vi "close.binary.refs.vi"(8 "error in":errorcluster, 11 "binary references":T1) -> (0 "error out":errorcluster)   [LabVIEW 2024, in "manager_daemon.lvclass"]
uses:
  manager_daemon.lvclass
  binary.references--cluster.ctl
  manager_daemon.lvclass/manager_daemon.ctl
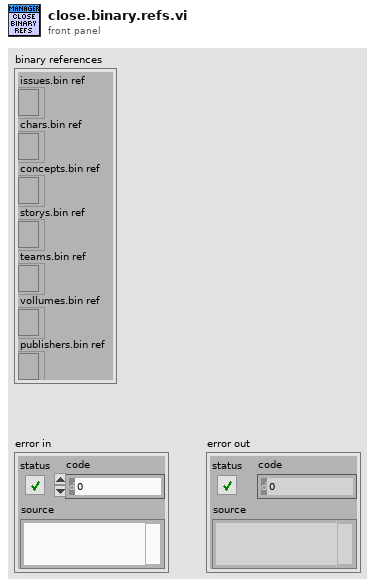
[diagram p1: front panel]
types:
  T1 = typedef "manager_daemon.lvclass/binary.references--cluster.ctl" = cluster{"issues.bin ref":refnum<file>, "chars.bin ref":refnum<file>, "concepts.bin ref":refnum<file>, "storys.bin ref":refnum<file>, "teams.bin ref":refnum<file>, "vollumes.bin ref":refnum<file>, "publishers.bin ref":refnum<file>}
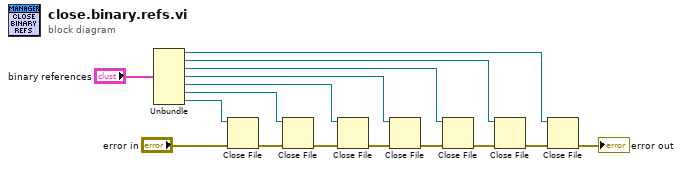
[diagram p0: block diagram]
diagram:
  n1 = Unbundle("binary references") -> ("issues.bin ref"=w3:refnum<file>, "chars.bin ref"=w4:refnum<file>, "concepts.bin ref"=w5:refnum<file>, "storys.bin ref"=w6:refnum<file>, "teams.bin ref"=w7:refnum<file>, "vollumes.bin ref"=w8:refnum<file>, "publishers.bin ref"=w15:refnum<file>)
  n2 = Close File(refnum=w15, error in="error in") -> (error out=w11:errorcluster)  [unwired: 1 out]
  n3 = Close File(refnum=w8, error in=w11) -> (error out=w14:errorcluster)  [unwired: 1 out]
  n4 = Close File(refnum=w7, error in=w14) -> (error out=w13:errorcluster)  [unwired: 1 out]
  n5 = Close File(refnum=w6, error in=w13) -> (error out=w10:errorcluster)  [unwired: 1 out]
  n6 = Close File(refnum=w5, error in=w10) -> (error out=w12:errorcluster)  [unwired: 1 out]
  n7 = Close File(refnum=w4, error in=w12) -> (error out=w9:errorcluster)  [unwired: 1 out]
  n8 = Close File(refnum=w3, error in=w9) -> (error out=→"error out":errorcluster)  [unwired: 1 out]
